vi "34_Basics of Stacked.vi"() -> ()   [LabVIEW 2018]
panel:
  out "Multiplication":dbl
  out "Subtraction":dbl
  out "Addition":dbl
  in  "Numeric 2":dbl
  in  "Numeric":dbl
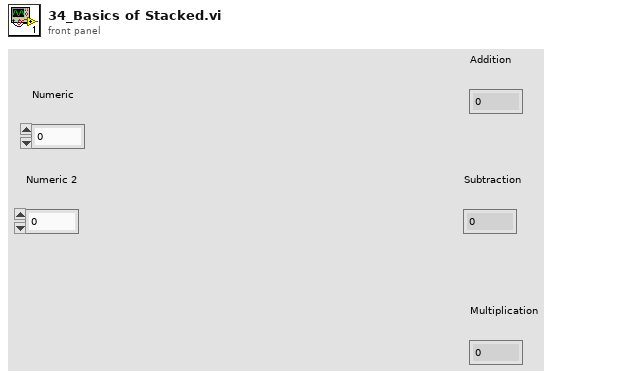
[diagram p1: front panel]
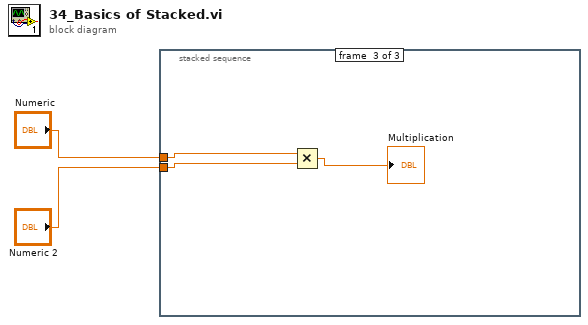
[diagram p0: block diagram]
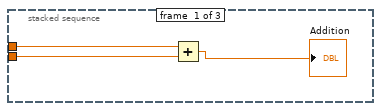
[diagram p2: hidden frame]
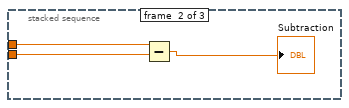
[diagram p3: hidden frame]
diagram:
  n1 = stacked-sequence {
    tunnel: "Numeric" -> [w5 w8 w11]
    tunnel: "Numeric 2" -> [w4 w7 w10]
    frame #0 {
      n2 = Add(x=w5, y=w4) -> (x+y=→"Addition":dbl)
    }
    frame #1 {
      n3 = Subtract(x=w8, y=w7) -> (x-y=→"Subtraction":dbl)
    }
    frame #2 {
      n4 = Multiply(x=w11, y=w10) -> (x*y=→"Multiplication":dbl)
    }
  }
